vi "Set-Point Driver.vi"   [LabVIEW 2013]
types:
  T1 = typedef "Semaphore RefNum" = refnum<k1>
  T2 = typedef "Sidecar Debug Queue.ctl" = refnum<queue>
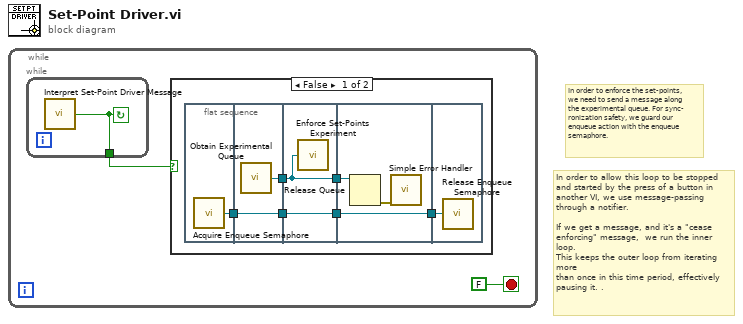
[diagram p0: block diagram]
diagram:
  # "In order to allow this loop to be stopped\nand started by the press of a button in \nanother VI, we use message-passing\nthrough a notifier. \n\nIf we get a message, and it's a \"cease \nenforcing\" message,  we run the inner loop.\nThis keeps the outer loop from iterating more\nthan once in this time period, effectively  \npausing it. ."
  # "In order to enforce the set-points,\nwe need to send a message along\nthe experimental queue. For sync-\nronization safety, we guard our \nenqueue action with the enqueue\nsemaphore."
  n1 = while {
    stop <- FALSE stop-if-true
    n2 = while {
      tunnel: [w3] -> w1
      stop <- w3 continue-if-true
      n3 = call "Interpret Set-Point Driver Message.vi"() -> ("Pause"=w3:bool)
    }
    n4 = case shown="False" w1 {
      frame False {
        n5 = flat-sequence {
          tunnel: [w10] -> w9
          tunnel: w9 -> [w12]
          tunnel: [w12] -> w8
          tunnel: [w11] -> w7
          tunnel: w8 -> [w14]
          tunnel: w7 -> [w13]
          tunnel: [w14] -> w6
          tunnel: [w13] -> w5
          tunnel: [w17] -> w4
          tunnel: w6 -> [w17]
          tunnel: w5 -> [w16]
          tunnel: w4 -> [w18]
          frame #0 {
            n6 = call "Acquire Enqueue Semaphore.vi"() -> ("Semaphore Reference"=w10:T1)
          }
          frame #1 {
            n7 = call "Obtain Experimental Queue.vi"() -> ("Queue"=w11:T2)
          }
          frame #2 {
            n8 = call "Enforce Set-Points Experiment.vi"("Experimental Queue"=w13) -> ()
          }
          frame #3 {
            n9 = Release Queue(queue=w16) -> (error out=w15:errorcluster)  [unwired: 2 in, 2 out]
            n10 = call <vilib>:"Simple Error Handler.vi"("error in (no error)"=w15) -> ()  [unwired: 4 in, 5 out]
          }
          frame #4 {
            n11 = call "Release Enqueue Semaphore.vi"("Semaphore Reference"=w18) -> ()
          }
        }
      }
      frame True {
      }
    }
  }
